vi "Close ROV.vi"(8 "error in (no error)":errorcluster, 11 "ROV in":refnum<class "ROV Host.lvclass">) -> (0 "error out":errorcluster)   [LabVIEW 2012, in "ROV Host.lvclass"]
doc: "This VI is simply used to close any resources or wrap up any loose ends utilized during the ROV session.\nRuffin"
uses:
  ROV Host.lvclass
  ROV Host.lvclass/ROV Host.ctl
  <vilib>/Utility/inputDevices.llb/closeJoystick.vi
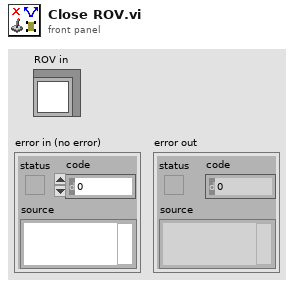
[diagram p1: front panel]
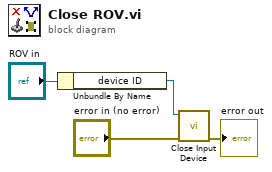
[diagram p0: block diagram]
diagram:
  n1 = Unbundle By Name("ROV in") -> ("device ID"=w1:refnum<k1>)
  n2 = call-poly <vilib>:"Close Input Device.vi"("error in (no error)"="error in (no error)", "device ID"=w1) -> ("error out"=→"error out":errorcluster)  [unwired: 8 in]
